vi "Read RP I-V Configuration.vi"(8 "error in (no error)":errorcluster, 11 "RP I-V in":refnum<class "RP I-V.lvclass">) -> (0 "error out":errorcluster, 2 "Configuration":T1 {"Recorder"."Rate" format="%#_8pHz"; "Recorder"."Post-trigger duration" format="%#_6ps"; "Recorder"."Pre-trigger duration" format="%#_6ps"; "Recorder"."Ranges" format="%#_6pV"; "I-V parameters"."Valhalla range" format="%#_6pA"; "I-V parameters"."Processing Delay" format="%dpts"; "I-V parameters"."Threshold" format="%#_6pV"; "I-V parameters"."Top  length" format="%dpts"; "I-V parameters"."Ramp length" format="%dpts"; "I-V parameters"."Baseline length" format="%dpts"; "I-V parameters"."Magnitude increment" format="%#_6pA"; "I-V parameters"."Start magnitude" format="%#_6pA"}, 3 "RP I-V out":refnum<class "RP I-V.lvclass">)   [LabVIEW 2016, in "RP I-V.lvclass"]
uses:
  RP I-V.lvclass
  C:/github/Measure_core/Template Module/Template Module.lvclass
  NHMFL_Core/Libraries/Red Pitaya/RP Core/Rep Pitaya I-V driver/RP I-V Configuration.ctl
  NHMFL_Core/Libraries/Instruments/Pulse Driver/Pusle Driver Configuration.ctl
  NHMFL_Core/Libraries/Red Pitaya/Waform generation/I-V parameters.ctl
  Measure_core/Template Module/Template Module.lvclass/Template Module.ctl
  Measure_core/Template Module/Read Configuration.vi
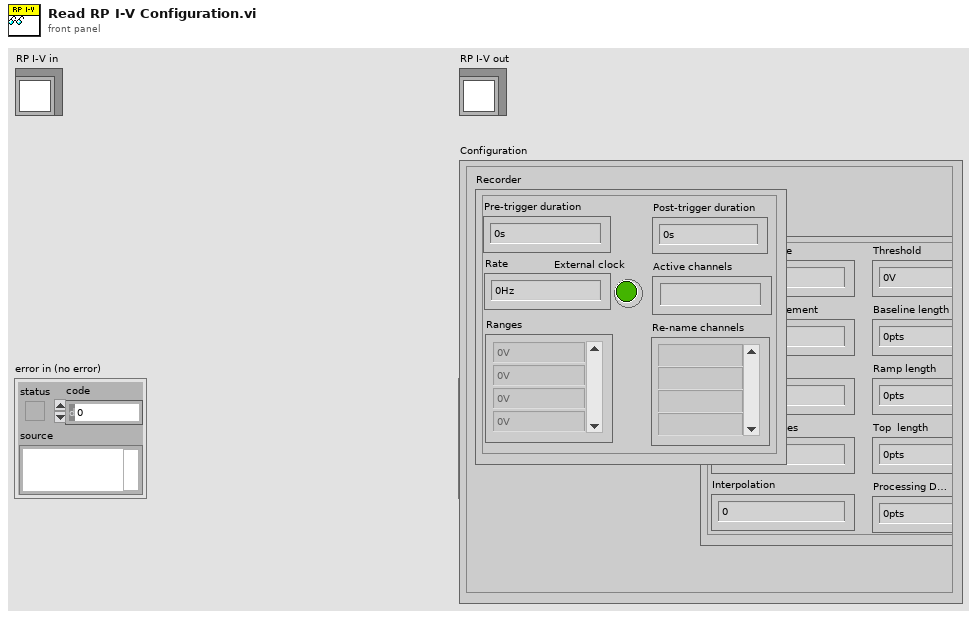
[diagram p1: front panel]
types:
  T1 = typedef "RP I-V Configuration.ctl" = cluster{"Recorder":T2, "I-V parameters":T3}
  T2 = typedef "Pusle Driver Configuration.ctl" = cluster{"Pre-trigger duration":dbl, "Post-trigger duration":dbl, "Rate":dbl, "Ranges":dbl[], "Re-name channels":string[], "Active channels":string, "External clock":bool}
  T3 = typedef "I-V parameters.ctl" = cluster{"Start magnitude":dbl, "Magnitude increment":dbl, "Number of pulses":i32, "Baseline length":i32, "Ramp length":i32, "Top  length":i32, "Threshold ":dbl, "Processing Delay":u16, "Valhalla range":dbl, "Interpolation":i32}
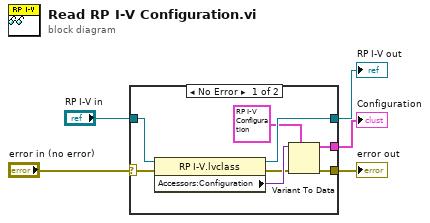
[diagram p0: block diagram]
diagram:
  n1 = case shown="No Error" "error in (no error)" {
    selector: "error in (no error)" -> [w7 w14]
    tunnel: [w6 w14] -> w2
    tunnel: [w10 w15] -> w5
    tunnel: "RP I-V in" -> [w11 w15]
    tunnel: [w8 _] -> w1
    frame No Error {
      n2 = property class="RP I-V.lvclass"(reference=w11, error in=w7) -> (reference out=w10:refnum<class "RP I-V.lvclass">, error out=w12:errorcluster, "Accessors:Configuration"=w13:variant)
      n3 = Variant To Data(error in=w12, type=T1 {"Recorder"={"Pre-trigger duration"=0.0, "Post-trigger duration"=0.0, "Rate"=0.0, "Ranges"=[], "Re-name channels"=[], "Active channels"="", "External clock"=FALSE}, "I-V parameters"={"Start magnitude"=0.0, "Magnitude increment"=0.0, "Number of pulses"=0, "Baseline length"=0, "Ramp length"=0, "Top  length"=0, "Threshold "=0.0, "Processing Delay"=0, "Valhalla range"=0.0, "Interpolation"=0}} ("Configuration"), Variant=w13) -> (data=w8:T1, error out=w6:errorcluster)
    }
    frame Error {
    }
  }
  "error out" <- w2
  "RP I-V out" <- w5
  "Configuration" <- w1
